vi "Configure TIE.vi"(8 "error in (no error)":errorcluster, 9 "Frequency (1 Hz)":dbl=1.0, 10 "Auto (T: On)":bool=TRUE, 11 "VISA resource name":refnum<visa-resource-name>) -> (0 "error out":errorcluster, 3 "VISA resource name out":refnum<visa-resource-name>)   [LabVIEW 2019, in "Pendulum CNT90.lvlib"]
doc: "Time Interval Error (TIE) measurement uses continuous time-stamping to observe slow phase shifts (wander) in nominally stable signals during extended periods of time. \nThe frequency of the signal to be checked can be either manually or automatically set. \n\n<B>Note:</B> VI is intended for use with CNT-91 only."
uses:
  Pendulum CNT90.lvlib
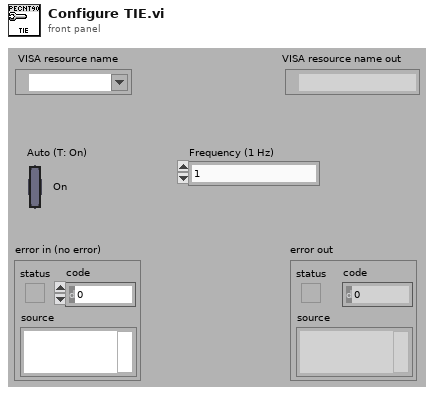
[diagram p1: front panel]
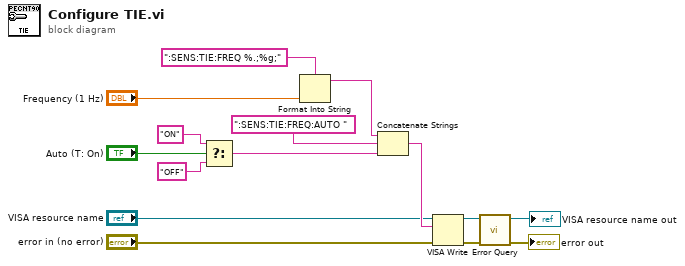
[diagram p0: block diagram]
diagram:
  n1 = Select(t="ON", s="Auto (T: On)", f="OFF") -> (s? t:f=w11:string)
  n2 = Format Into String(format string=":SENS:TIE:FREQ %.;%g;" ("Attenuation Command"), "Frequency (1 Hz)") -> (resulting string=w13:string)  [unwired: 2 in, 1 out]
  n3 = Concatenate Strings(w13, ":SENS:TIE:FREQ:AUTO ", w11) -> (w7:string)
  n4 = VISA Write(VISA resource name="VISA resource name", write buffer=w7, error in (no error)="error in (no error)") -> (VISA resource name out=w3:refnum<visa-resource-name>, error out=w4:errorcluster)  [unwired: 1 out]
  n5 = call "Error Query.vi"("error in (no error)"=w4, "VISA resource name"=w3) -> ("error out"=→"error out":errorcluster, "VISA resource name out"=→"VISA resource name out":refnum<visa-resource-name>)  [unwired: 6 in, 2 out]
